vi "uObserver_Publish_Event.vi"(8 "error in (no error)":errorcluster, 10 "uMsg":refnum<class "uMsg.lvclass">, 11 "uObserver in":refnum<class "uObserver.lvclass">) -> (0 "error out":errorcluster, 3 "uObserver out":refnum<class "uObserver.lvclass">)   [LabVIEW 2021, in "uFramework_pack_uActor.lvlib" / "uObserver.lvclass"]
doc: "Publish an event to the observed broker conforming to the Observer's publishing policy.\nFor optimal performance in high-throughput streaming applications, make sure to set a valid timestamp when creating the message to be published."
uses:
  uObserver.lvclass
  uObserver.lvclass/uObserver.ctl
  Bin/uFramework.lvlibp/uClient_Publisher/uClient_Publisher.lvclass
  Bin/uFramework.lvlibp/uMsg/uMsg.lvclass
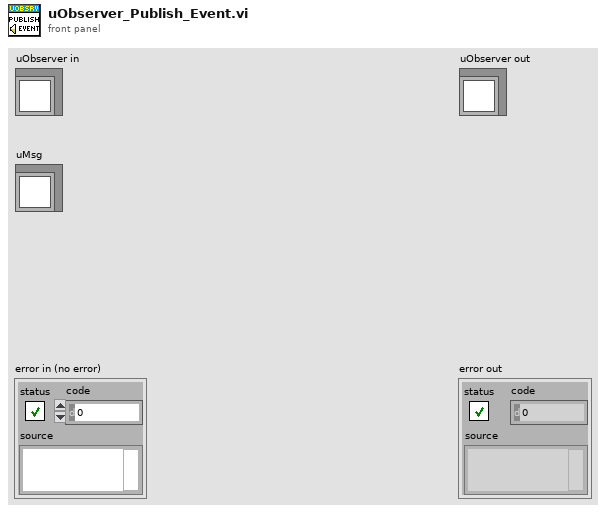
[diagram p1: front panel]
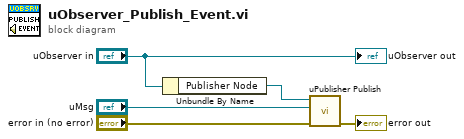
[diagram p0: block diagram]
diagram:
  n1 = Unbundle By Name("uObserver in") -> ("Publisher Node"=w1:refnum<class "uClient_Publisher.lvclass">)
  n2 = call "uPublisher Publish.vi"("error in (no error)"="error in (no error)", "uMsg"="uMsg", "uClient_Publisher in"=w1) -> ("error out"=→"error out":errorcluster)  [unwired: 7 in, 1 out]
  "uObserver out" <- "uObserver in"
